vi "com port send response test cluster.vi"(0 "VISA Send port":refnum<visa-resource-name>, 5 "AT CMD List":T1, 9 "Log in":string, 11 "error in (no error)":errorcluster, 12 "PassFail_In":bool=TRUE) -> (4 "VISA Send port out":refnum<visa-resource-name>, 6 "Response":string, 10 "Log out":string, 14 "PassFail_Out":bool, 15 "error out":errorcluster)   [LabVIEW 2013]
uses:
  AT cmd list.ctl
  Test Support VI/String compare type.ctl
panel:
  out "Bytes at port":u32
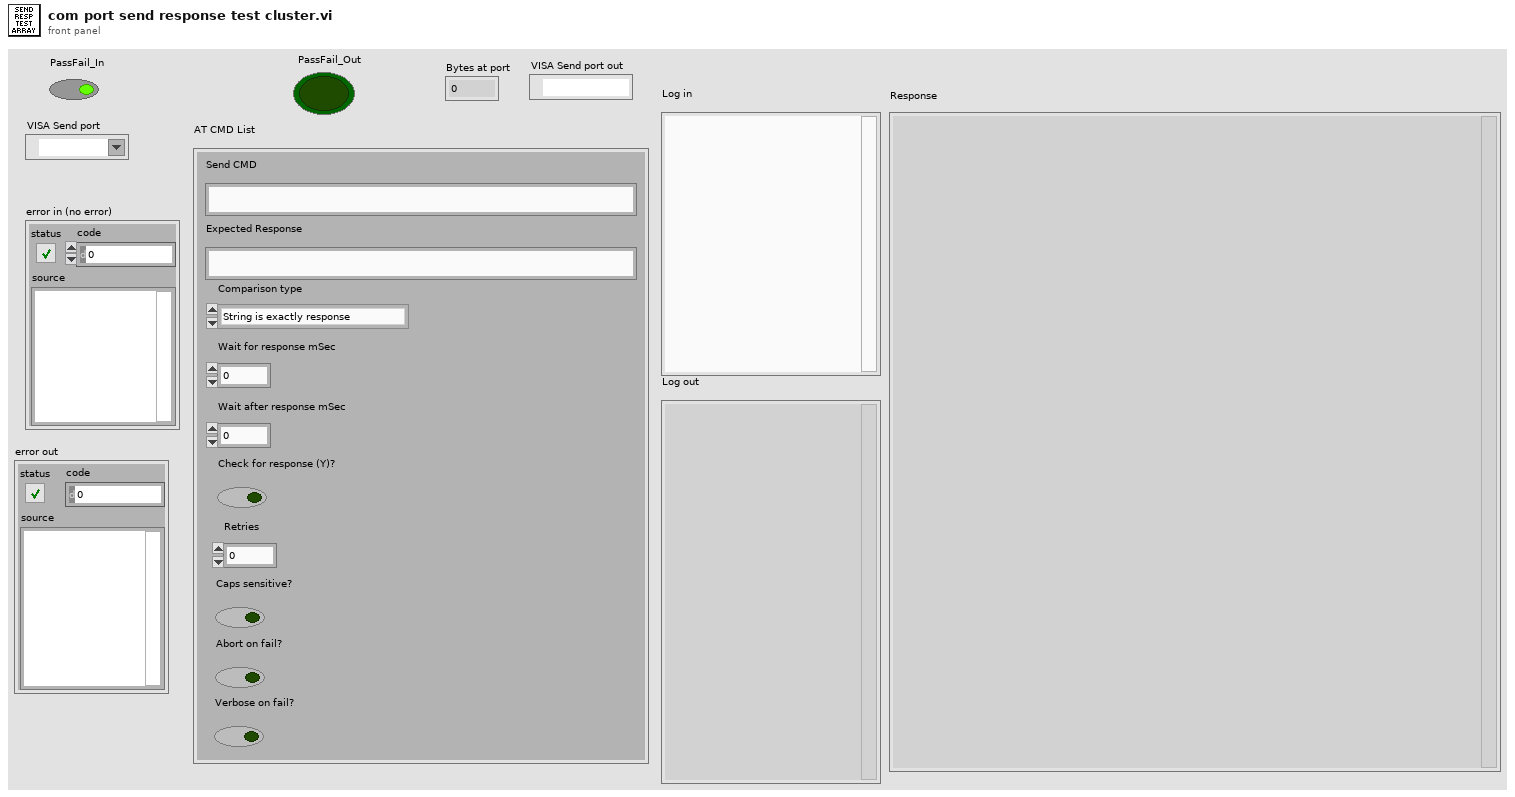
[diagram p1: front panel]
types:
  T1 = typedef "AT cmd list.ctl" = cluster{"Send CMD":string, "Expected Response":string, "Comparison type":T2, "Wait for response mSec":dbl, "Wait after response mSec":dbl, "Check for response (Y)?":bool, "Retries":dbl, "Caps sensitive?":bool, "Abort on fail?":bool, "Verbose on fail?":bool}
  T2 = typedef "String compare type.ctl" = enum16{"String is exactly response", "String in response somewhere", "String not in response"}
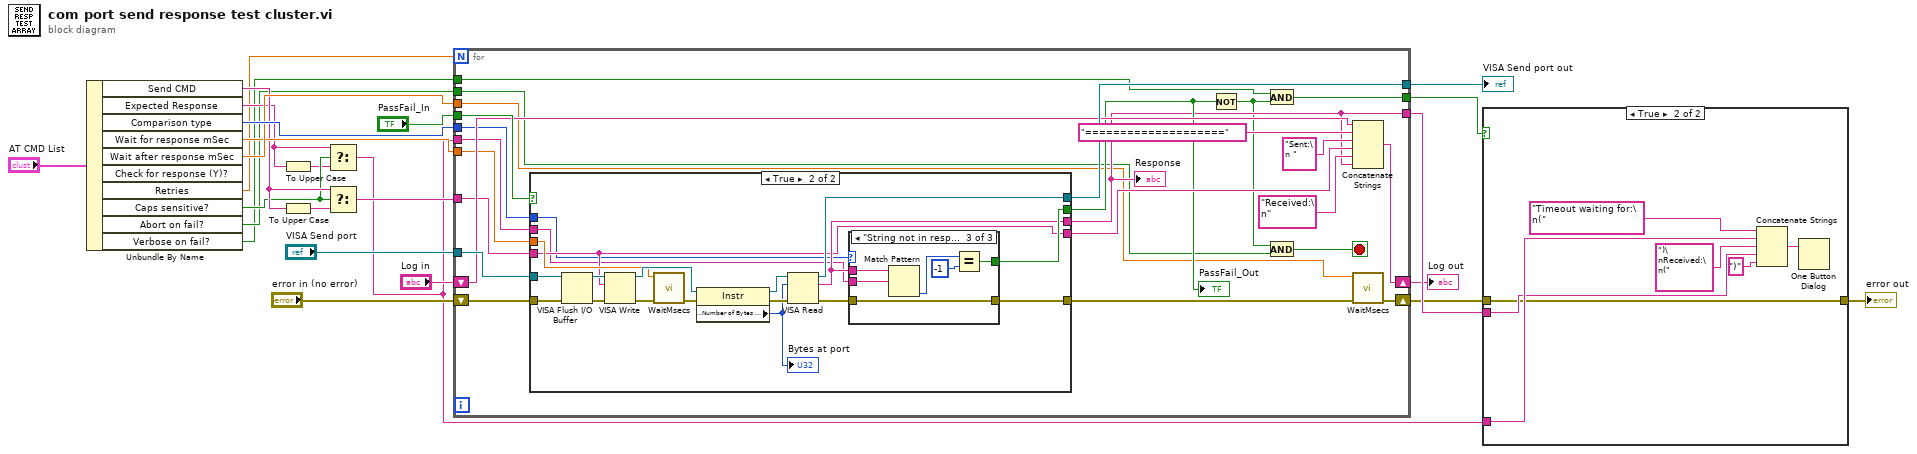
[diagram p0: block diagram]
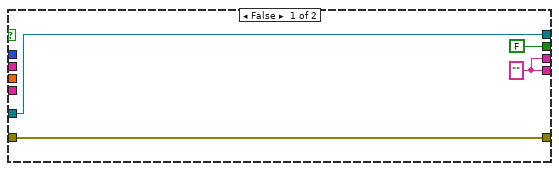
[diagram p2: hidden frame]
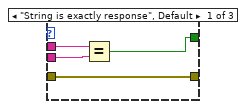
[diagram p3: hidden frame]
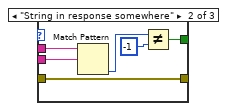
[diagram p4: hidden frame]
diagram:
  n1 = Unbundle By Name("AT CMD List") -> ("Send CMD"=w11:string, "Expected Response"=w7:string, "Comparison type"=w15:T2, "Wait for response mSec"=w13:dbl, "Wait after response mSec"=w14:dbl, "Retries"=w5:dbl, "Caps sensitive?"=w9:bool, "Abort on fail?"=w4:bool, "Verbose on fail?"=w1:bool)  [unwired: 1 out]
  n2 = To Upper Case(1:w7) -> (0:w8:string)
  n3 = To Upper Case(1:w11) -> (0:w12:string)
  n4 = Select(t=w7, s=w9, f=w8) -> (s? t:f=w6:string)
  n5 = Select(t=w11, s=w9, f=w12) -> (s? t:f=w10:string)
  n6 = for {
    N: w5 -> [_]
    tunnel: "VISA Send port" -> [w48]
    tunnel: "PassFail_In" -> [w46]
    tunnel: [w45] -> w21
    tunnel: [w37] -> w19
    tunnel: [w36] -> w18
    tunnel: w15 -> [w35]
    tunnel: w14 -> [w34]
    tunnel: w13 -> [w33]
    tunnel: w1 -> [w32]
    tunnel: w10 -> [w31]
    tunnel: w6 -> [w30]
    tunnel: w4 -> [w29]
    shift-right: [w26] -> w3
    shift-left: "Log in" -> [w43]
    shift-right: [w25] -> w2
    shift-left: "error in (no error)" -> [w47]
    stop <- w27 stop-if-true
    n7 = case shown="True" w46 {
      tunnel: [FALSE w64] -> w38
      tunnel: w48 -> [w50 w61]
      tunnel: [w51 w60] -> w44
      tunnel: w47 -> [w51 w63]
      tunnel: [w50 w58] -> w45
      tunnel: w33 -> [_ w57]
      tunnel: w31 -> [_ w55]
      tunnel: [w49 w56] -> w36
      tunnel: [w49 w55] -> w42
      tunnel: w30 -> [_ w54]
      tunnel: w35 -> [_ w53]
      frame False {
        w49 = "" ("read buffer")
      }
      frame True {
        n8 = VISA Flush I/O Buffer(VISA resource name=w61, error in (no error)=w63) -> (VISA resource name out=w70:refnum<visa-resource-name>, error out=w71:errorcluster)  [unwired: 1 in]
        n9 = VISA Write(VISA resource name=w70, write buffer=w55, error in (no error)=w71) -> (VISA resource name out=w59:refnum<visa-resource-name>, error out=w69:errorcluster)  [unwired: 1 out]
        n10 = call "WaitMsecs.vi"("error in (no error)"=w69, "Wait Msecs"=w57) -> ("error out"=w68:errorcluster)  [unwired: 9 in]
        n11 = property class="Instr"(reference=w59, error in=w68) -> (reference out=w65:refnum<visa-resource-name>, error out=w67:errorcluster, "Serial Settings:Number of Bytes at Serial Port"=w66:u32)
        "Bytes at port" <- w66
        n12 = VISA Read(VISA resource name=w65, byte count=w66, error in (no error)=w67) -> (VISA resource name out=w58:refnum<visa-resource-name>, read buffer=w56:string, error out=w62:errorcluster)  [unwired: 1 out]
        n13 = case shown="\"String not in response\"" w53 {
          tunnel: w56 -> [w75 w81 w85]
          tunnel: w62 -> [w72 w76 w82]
          tunnel: w54 -> [w74 w80 w84]
          tunnel: [w73 w77 w83] -> w64
          tunnel: [w72 w76 w82] -> w60
          frame "String is exactly response", Default {
            n14 = Equal?(x=w75, y=w74) -> (x = y?=w73:bool)
          }
          frame "String in response somewhere" {
            n15 = Match Pattern(string=w81, regular expression=w80) -> (offset past match=w79:i32)  [unwired: 1 in, 3 out]
            n16 = Not Equal?(x=w79, y=-1) -> (x != y?=w77:bool)
          }
          frame "String not in response" {
            n17 = Match Pattern(string=w85, regular expression=w84) -> (offset past match=w87:i32)  [unwired: 1 in, 3 out]
            n18 = Equal?(x=w87, y=-1) -> (x = y?=w83:bool)
          }
        }
      }
    }
    "PassFail_Out" <- w38
    "Response" <- w36
    n19 = Not(x=w38) -> (.not. x?=w28:bool)
    n20 = And(x=w32, y=w28) -> (x .and. y?=w37:bool)
    n21 = And(x=w28, y=w29) -> (x .and. y?=w27:bool)
    n22 = Concatenate Strings(w43, "====================" ("string"), "Sent:\n " ("string"), w42, "Received:\n" ("string"), w36) -> (w26:string)
    n23 = call "WaitMsecs.vi"("error in (no error)"=w44, "Wait Msecs"=w34) -> ("error out"=w25:errorcluster)  [unwired: 9 in]
  }
  "VISA Send port out" <- w21
  "Log out" <- w3
  n24 = case shown="True" w19 {
    tunnel: w6 -> [_ w94]
    tunnel: w18 -> [_ w92]
    tunnel: [w88 w89] -> w17
    tunnel: w2 -> [w88 w89]
    frame False {
    }
    frame True {
      n25 = Concatenate Strings("Timeout waiting for:\n(" ("string"), w94, ")\nReceived:\n(" ("string"), w92, ")" ("string")) -> (w90:string)
      n26 = One Button Dialog(message=w90) -> ()  [unwired: 1 in, 1 out]
    }
  }
  "error out" <- w17
